vi "read_set_preregistration_data_msg.vi"(8 "error_in":errorcluster, 11 "command":string) -> (0 "error_out":errorcluster, 3 "preregistration_data":T1 {"Starting serial number" format="%#_11g"})   [LabVIEW 2018]
uses:
  controls/preregistration_data.ctl
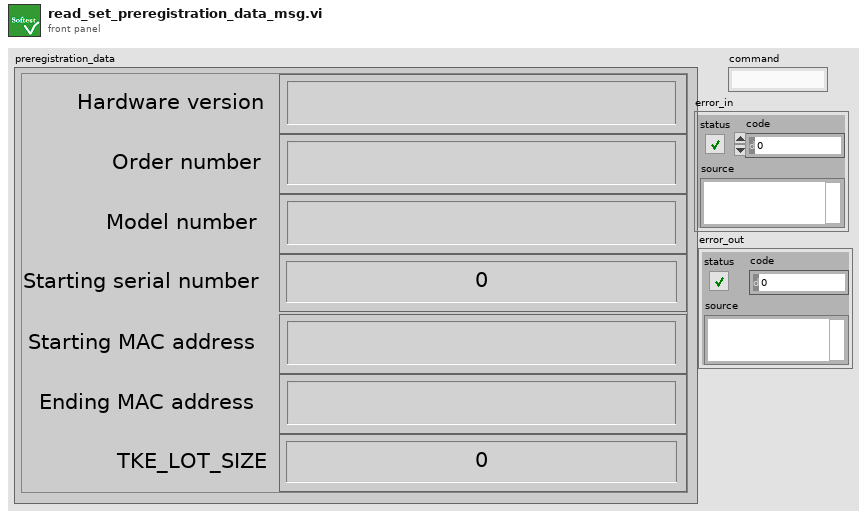
[diagram p1: front panel]
types:
  T1 = typedef "preregistration_data.ctl" = cluster{"Hardware version":string, "Order number":string, "Model number":string, "Starting serial number":i32, "Starting MAC address":string, "Ending MAC address":string, "TKE_LOT_SIZE":i32}
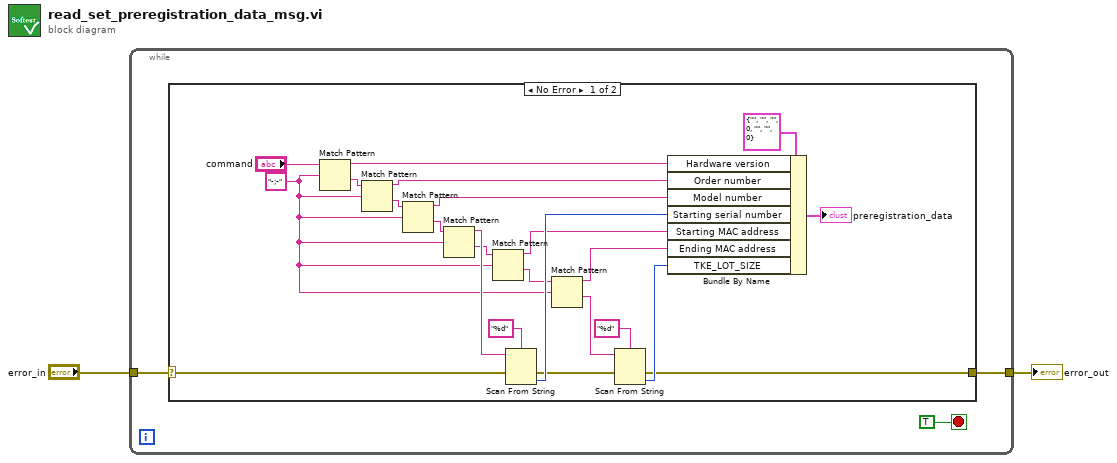
[diagram p0: block diagram]
diagram:
  n1 = while {
    tunnel: "error_in" -> [w4]
    tunnel: [w3] -> w1
    stop <- TRUE stop-if-true
    n2 = case shown="No Error" w4 {
      selector: w4 -> [w18 w29]
      tunnel: [w6 w29] -> w3
      frame No Error {
        w13 = "-;-" ("string")
        n3 = Match Pattern(string="command", regular expression=w13) -> (before substring=w27:string, after substring=w26:string)  [unwired: 1 in, 2 out]
        n4 = Match Pattern(string=w26, regular expression=w13) -> (before substring=w23:string, after substring=w22:string)  [unwired: 1 in, 2 out]
        n5 = Match Pattern(string=w22, regular expression=w13) -> (before substring=w21:string, after substring=w20:string)  [unwired: 1 in, 2 out]
        n6 = Match Pattern(string=w20, regular expression=w13) -> (before substring=w19:string, after substring=w15:string)  [unwired: 1 in, 2 out]
        n7 = Match Pattern(string=w15, regular expression=w13) -> (before substring=w14:string, after substring=w12:string)  [unwired: 1 in, 2 out]
        n8 = Scan From String(format string="%d", input string=w19, error in=w18) -> (error out=w10:errorcluster, output 1=w16:i32)  [unwired: 2 in, 2 out]
        n9 = Match Pattern(string=w12, regular expression=w13) -> (before substring=w11:string, after substring=w8:string)  [unwired: 1 in, 2 out]
        n10 = Scan From String(format string="%d", input string=w8, error in=w10) -> (error out=w6:errorcluster, output 1=w7:i32)  [unwired: 2 in, 2 out]
        n11 = Bundle By Name(cluster=T1 {"Hardware version"="", "Order number"="", "Model number"="", "Starting serial number"=0, "Starting MAC address"="", "Ending MAC address"="", "TKE_LOT_SIZE"=0} ("preregistration_data"), "Hardware version"=w27, "Order number"=w23, "Model number"=w21, "Starting serial number"=w16, "Starting MAC address"=w14, "Ending MAC address"=w11, "TKE_LOT_SIZE"=w7) -> (→"preregistration_data":T1)
      }
      frame Error {
      }
    }
  }
  "error_out" <- w1
